vi "1D DBL Array_Sort and Delete Repeating Sells.vi"(2 "1D DBL Array.In":dbl[](array[numeric])) -> (6 "1D DBL Array.Out":dbl[](array[numeric]))   [LabVIEW 2020]
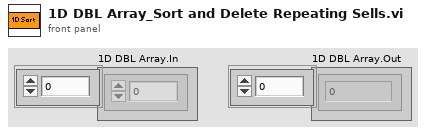
[diagram p1: front panel]
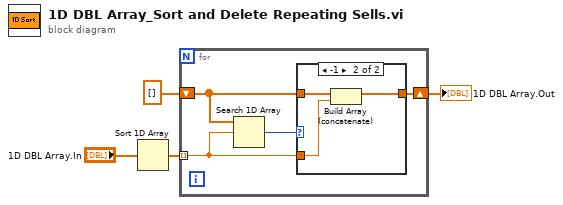
[diagram p0: block diagram]
diagram:
  n1 = Sort 1D Array(array="1D DBL Array.In") -> (sorted array=w2:dbl[])
  n2 = for {
    tunnel: w2 -> [w6] mode=indexing
    shift-right: [w5] -> w4
    shift-left: dbl[] [] ("sorted array") -> [w7]
    n3 = Search 1D Array(1D array=w7, element=w6) -> (index of element=w8:i32)  [unwired: 1 in]
    n4 = case shown="-1" w8 {
      tunnel: w7 -> [w9 w12]
      tunnel: w6 -> [_ w11]
      tunnel: [w9 w10] -> w5
      frame 0, Default {
      }
      frame -1 {
        n5 = Build Array (concatenate)(w12, w11) -> (w10:dbl[])
      }
    }
  }
  "1D DBL Array.Out" <- w4
